vi "DigitalInstrument_CallInitializeMeasurementLinkSessionWithCreateBehavior_RemoteSessionCreated.vi"(8 "error in":errorcluster) -> (0 "error out":errorcluster, 2 "result":string, 3 "pass":bool)   [LabVIEW 2020, in "MeasurementServerTests.lvlib"]
uses:
  MeasurementServerTests.lvlib
  Runtime/MeasurementLink Instrument/IInstrument/Initialize Session Behavior.ctl
  Runtime/MeasurementLink Instrument/IInstrument/IInstrument.lvclass
  Runtime/MeasurementLink niDigital/Instrument/Instrument.lvclass
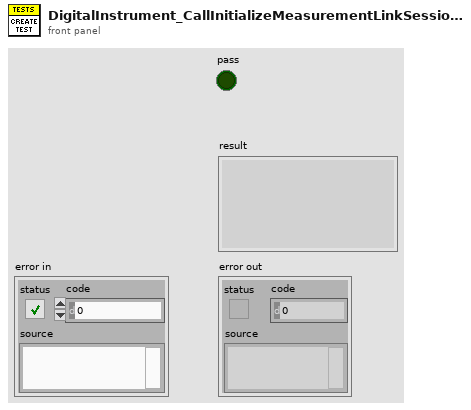
[diagram p1: front panel]
types:
  T1 = typedef "MeasurementLink Instrument.lvlib/IInstrument.lvclass/Remote Connection Options.ctl" = cluster{"session name":string, "address":string, "port":u32}
  T2 = typedef "MeasurementLink Instrument.lvlib/IInstrument.lvclass/Initialize Session Behavior.ctl" = enum16{"Create Session", "Attach Session"}
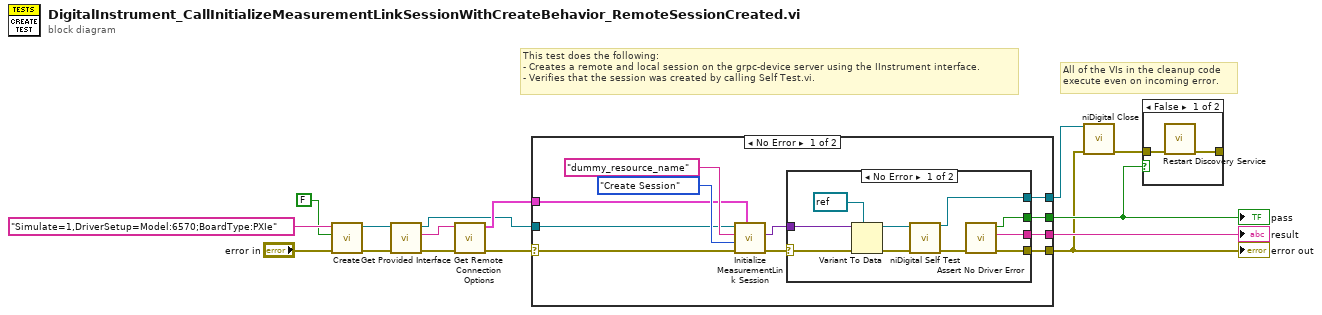
[diagram p0: block diagram]
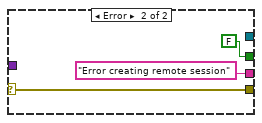
[diagram p2: hidden frame]
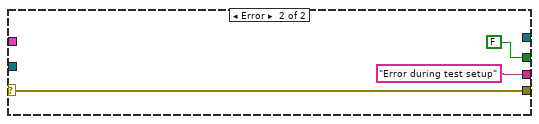
[diagram p3: hidden frame]
diagram:
  # "All of the VIs in the cleanup code\nexecute even on incoming error."
  # "This test does the following:\n- Creates a remote and local session on the grpc-device server using the IInstrument interface.\n- Verifies that the session was created by calling Self Test.vi."
  n1 = call "Create.vi"("error in"="error in", "reset"=FALSE, "option string"="Simulate=1,DriverSetup=Model:6570;BoardType:PXIe") -> ("error out"=w1:errorcluster, "instrument out"=w2:refnum<class "Instrument.lvclass">)  [unwired: 7 in]
  n2 = call-dynamic "Get Provided Interface.vi"("error in"=w1, "instrument in"=w2) -> ("error out"=w13:errorcluster, "provided interface"=w14:string, "instrument out"=w10:refnum<class "Instrument.lvclass">)  [unwired: 7 in]
  n3 = call "Get Remote Connection Options.vi"("error in"=w13, "provided interface"=w14) -> ("error out"=w12:errorcluster, "remote connection options"=w11:T1)  [unwired: 8 in]
  n4 = case shown="No Error" w12 {
    selector: w12 -> [w19 w40]
    tunnel: [w25 w40] -> w6
    tunnel: [w26 FALSE] -> w7
    tunnel: [w24 "Error during test setup" ("f")] -> w15
    tunnel: w11 -> [w18 _]
    tunnel: w10 -> [w17 _]
    tunnel: [w16 _] -> w9
    frame No Error {
      n5 = call-dynamic "Initialize MeasurementLink Session.vi"("remote connection options"=w18, "error in"=w19, "initialize session behavior"=Initialize_Session_Behavior."Create Session", "resource name"="dummy_resource_name", "instrument in"=w17) -> ("error out"=w22:errorcluster, "session out"=w23:variant)  [unwired: 4 in, 1 out]
      n6 = case shown="No Error" w22 {
        selector: w22 -> [w33 w38]
        tunnel: [w36 FALSE] -> w26
        tunnel: [w31 w38] -> w25
        tunnel: [w35 "Error creating remote session"] -> w24
        tunnel: w23 -> [w34 _]
        tunnel: [w30 _] -> w16
        frame No Error {
          n7 = Variant To Data(error in=w33, type=refnum<k15> refnum ("instrument handle in"), Variant=w34) -> (data=w27:refnum<k15>, error out=w32:errorcluster)
          n8 = call <instrlib>:"niDigital Self Test.vi"("instrument handle in"=w27, "error in"=w32) -> ("instrument handle out"=w30:refnum<k15>, "error out"=w29:errorcluster)  [unwired: 10 in, 2 out]
          n9 = call "Assert No Driver Error.vi"("error in"=w29) -> ("error out"=w31:errorcluster, "result"=w35:string, "pass?"=w36:bool)  [unwired: 8 in]
        }
        frame Error {
        }
      }
    }
    frame Error {
    }
  }
  "error out" <- w6
  "pass" <- w7
  "result" <- w15
  n10 = call <instrlib>:"niDigital Close.vi"("instrument handle"=w9, "error in"=w6) -> ("error out"=w8:errorcluster)  [unwired: 13 in]
  n11 = case shown="False" w7 {
    tunnel: w8 -> [w44 _]
    tunnel: [w43 _] -> _
    frame False {
      n12 = call "Restart Discovery Service.vi"("error in"=w44) -> ("error out"=w43:errorcluster)  [unwired: 10 in]
    }
    frame True {
    }
  }
